vi "for_loop.vi"() -> ()   [LabVIEW 2014]
panel:
  out "Inner Loop #":i32
  out "Result":dbl
  out "Outer Loop #":i32
  in  "Array":dbl[][](array[numeric])=[[1.0, 2.0, 3.0], [4.0, 5.0, 6.0], [7.0, 8.0, 9.0]]
  # "Display Every Element in the 2D Array"
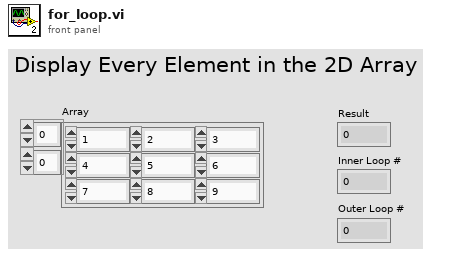
[diagram p1: front panel]
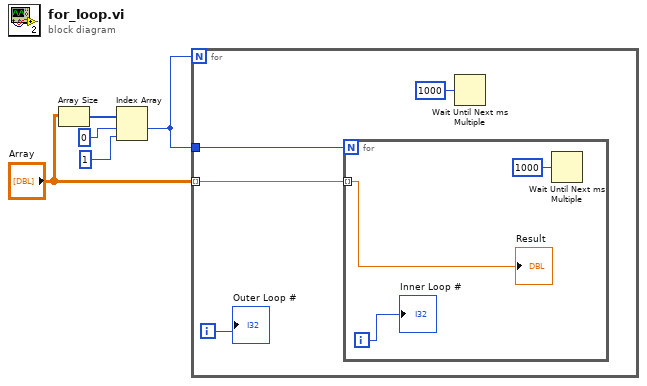
[diagram p0: block diagram]
diagram:
  n1 = Array Size(array="Array") -> (size(s)=w3:i32[])
  n2 = Index Array(array=w3, index #1=0 ("index"), index #2=1 ("index")) -> (element #1=w1:i32)  [unwired: 1 out]
  n3 = for {
    N: w1 -> [_]
    tunnel: "Array" -> [w6] mode=indexing
    tunnel: w1 -> [w7]
    i -> [w9]
    n4 = for {
      N: w7 -> [_]
      tunnel: w6 -> [w10] mode=indexing
      i -> [w11]
      n5 = Wait Until Next ms Multiple(millisecond multiple=u32 1000) -> ()  [unwired: 1 out]
      "Result" <- w10
      "Inner Loop #" <- w11
    }
    n6 = Wait Until Next ms Multiple(millisecond multiple=u32 1000) -> ()  [unwired: 1 out]
    "Outer Loop #" <- w9
  }
